vi "Test4-C.vi"(11 "Params":string[][](array[string])) -> ()   [LabVIEW 2017]
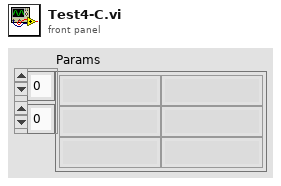
[diagram p1: front panel]
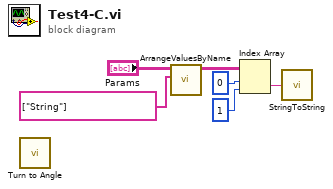
[diagram p0: block diagram]
diagram:
  n1 = call "Turn to Angle.vi"() -> ()  [unwired: 15 in, 1 out]
  n2 = call "ArrangeValuesByName.vi"("Names"=string[] ["String"], "Names/Values in"="Params") -> ("Names/Values Out"=w5:string[][])  [unwired: 9 in]
  n3 = Index Array(array=w5, index (row)=0, index (col)=1) -> (element=w1:string)
  n4 = call "StringToString.vi"("String"=w1) -> ()  [unwired: 1 out]
